vi "Pausable Timer.vi"(5 "Timer Mode":T1=enum."Read", 6 "Force Pause?":bool, 7 "Force Initialise?":bool, 8 "Error In":errorcluster, 10 "Desired Time (S)":dbl) -> (0 "Error Out":errorcluster, 1 "Time Up?":bool, 2 "Elapsed Time (S)":dbl)   [LabVIEW 2016]
doc: "A Pauseable Timer (FGV) based around the Get Time(ms) function.\nTimer sould be Initialised using the Timer Mode 'Initialise' or by setting the 'Force Initialise' boolean True on first call.\n\nTimer can be Paused either by using the Timer Mode 'Pause' or by setting the 'Force Pause' boolean True.\n\nThe Timer Mode 'Read' will resume from a Pause (assuming 'Force Pause' is False)\n\nD.Readman 7/2/2014"
uses:
  Timer Mode.ctl
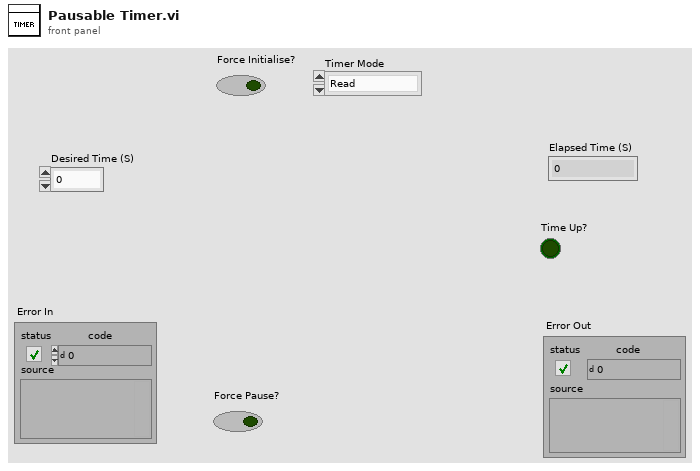
[diagram p1: front panel]
types:
  T1 = typedef "Timer Mode.ctl" = enum16{"Initialise", "Read", "Pause"}
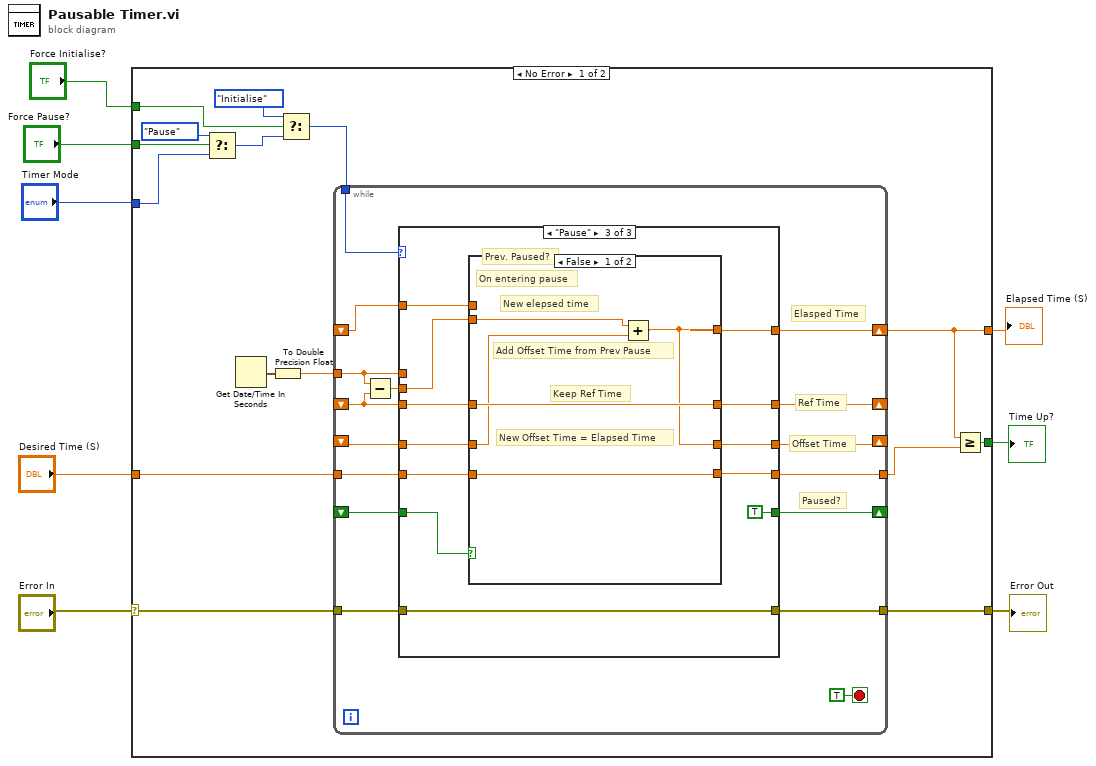
[diagram p0: block diagram]
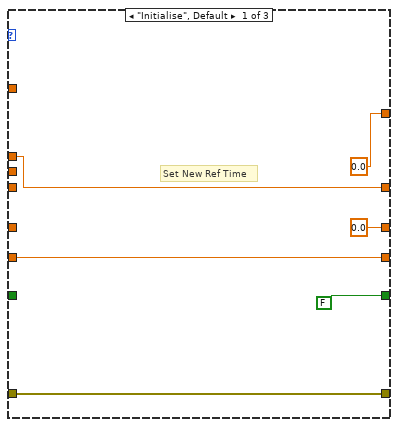
[diagram p2: hidden frame]
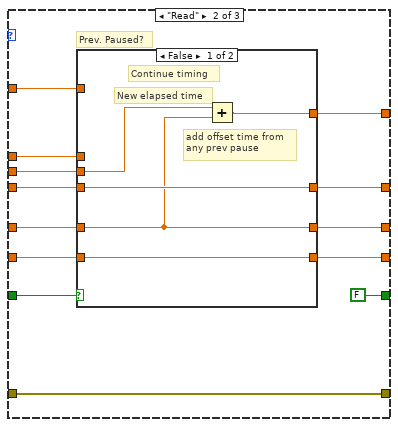
[diagram p3: hidden frame]
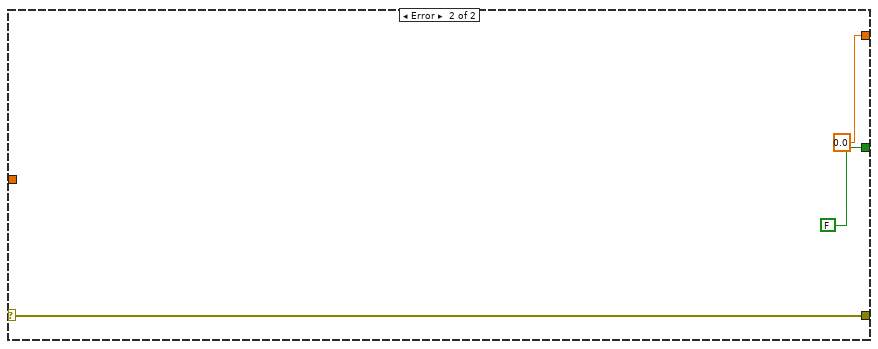
[diagram p6: hidden frame]
diagram:
  n1 = case shown="No Error" "Error In" {
    selector: "Error In" -> [w23 w90]
    tunnel: [w22 w90] -> w7
    tunnel: [w18 FALSE ("Time Up?")] -> w6
    tunnel: [w17 0.0 ("Elapsed Time (S)")] -> w5
    tunnel: "Timer Mode" -> [w14 _]
    tunnel: "Desired Time (S)" -> [w20 _]
    tunnel: "Force Pause?" -> [w15 _]
    tunnel: "Force Initialise?" -> [w9 _]
    frame No Error {
      n2 = Select(t=Timer_Mode."Pause" ("Timer Mode 2"), s=w15, f=w14) -> (s? t:f=w12:T1)
      n3 = Get Date/Time In Seconds() -> (seconds since 1Jan1904=w21:timestamp)
      n4 = To Double Precision Float(number=w21) -> (double precision float=w19:dbl)
      n5 = Select(t=Timer_Mode."Initialise", s=w9, f=w12) -> (s? t:f=w11:T1)
      n6 = while {
        tunnel: w23 -> [w38]
        tunnel: [w37] -> w22
        tunnel: w11 -> [w36]
        shift-right: [w34] -> _
        shift-left: _ -> [w25]
        tunnel: w20 -> [w35]
        tunnel: w19 -> [w26]
        tunnel: [w32] -> w16
        shift-right: [w31] -> _
        shift-left: _ -> [w28]
        shift-right: [w30] -> _
        shift-left: _ -> [w27]
        shift-right: [w33] -> w17
        shift-left: _ -> [w29]
        stop <- TRUE stop-if-true
        # "Elasped Time"
        # "Paused?"
        # "Offset Time"
        # "Ref Time"
        n7 = Subtract(x=w26, y=w25) -> (x-y=w24:dbl)
        n8 = case shown="\"Pause\"" w36 {
          tunnel: w38 -> [w45 w58 w77]
          tunnel: [w45 w58 w77] -> w37
          tunnel: [w43 w52 w70] -> w34
          tunnel: [w44 w48 w71] -> w32
          tunnel: w35 -> [w44 w49 w72]
          tunnel: w25 -> [_ w53 w69]
          tunnel: w26 -> [w43 w47 _]
          tunnel: [0.0 w54 w75] -> w33
          tunnel: [0.0 w50 w73] -> w31
          tunnel: [FALSE FALSE TRUE] -> w30
          tunnel: w29 -> [_ w46 w68]
          tunnel: w28 -> [_ w51 w67]
          tunnel: w27 -> [_ w56 w76]
          tunnel: w24 -> [_ w55 w74]
          frame "Initialise", Default {
            # "Set New Ref Time"
          }
          frame "Read" {
            # "Prev. Paused?"
            n9 = case shown="False" w56 {
              tunnel: w55 -> [w60 _]
              tunnel: [w61 w64] -> w54
              tunnel: w53 -> [w63 _]
              tunnel: [w63 w66] -> w52
              tunnel: w51 -> [w59 w64]
              tunnel: [w59 w64] -> w50
              tunnel: w49 -> [w62 w65]
              tunnel: [w62 w65] -> w48
              tunnel: w47 -> [_ w66]
              tunnel: w46 -> [_ _]
              frame False {
                # "add offset time from\nany prev pause"
                # "New elapsed time"
                # "Continue timing"
                n10 = Add(x=w60, y=w59) -> (x+y=w61:dbl)
              }
              frame True {
                # "Elapsed Time = Offset Time"
                # "Keep Offset time set while paused"
                # "New Ref Time"
                # "Restart the timer after pause"
              }
            }
          }
          frame "Pause" {
            # "Prev. Paused?"
            n11 = case shown="False" w76 {
              tunnel: w74 -> [w79 _]
              tunnel: [w81 w87] -> w75
              tunnel: [w81 w85] -> w73
              tunnel: w72 -> [w83 w84]
              tunnel: [w83 w84] -> w71
              tunnel: [w82 w86] -> w70
              tunnel: w69 -> [w82 w86]
              tunnel: w68 -> [_ w87]
              tunnel: w67 -> [w80 w85]
              frame False {
                # "Add Offset Time from Prev Pause"
                # "Keep Ref Time"
                # "New Offset Time = Elapsed Time"
                # "On entering pause"
                # "New elepsed time"
                n12 = Add(x=w79, y=w80) -> (x+y=w81:dbl)
              }
              frame True {
                # "Keep same offset time"
                # "Keep same ref time"
                # "Keep same elapsed time"
                # "On remaining pause"
              }
            }
          }
        }
      }
      n13 = Greater Or Equal?(x=w17, y=w16) -> (x >= y?=w18:bool)
    }
    frame Error {
    }
  }
  "Error Out" <- w7
  "Time Up?" <- w6
  "Elapsed Time (S)" <- w5
